vi "Write Teller.vi"(7 "Msg in":refnum<class "Msg.lvclass">, 10 "Teller":T1 {"Absolute Time" format="%<%x %.3X>T"}) -> (5 "Msg out":refnum<class "Msg.lvclass">)   [LabVIEW 2020, in "jettl.lvlib"]
uses:
  jettl.lvlib
  Msg/Msg.lvclass
  Teller Metadata/Teller Metadata.lvclass
  Msg Input/Msg Input.lvclass
  Teller.ctl
  Relation.ctl
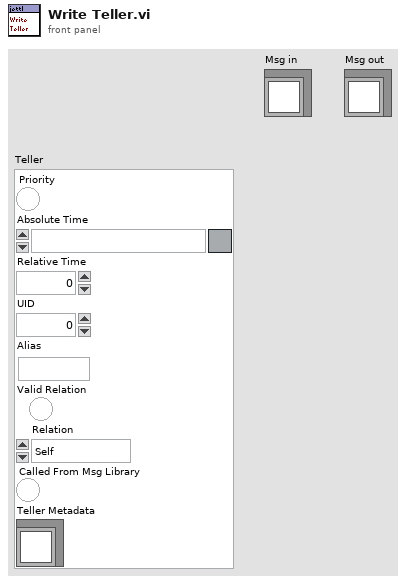
[diagram p1: front panel]
types:
  T1 = typedef "jettl.lvlib/Teller.ctl" = cluster{"Priority":bool, "Absolute Time":timestamp, "Relative Time":dbl, "UID":i32, "Alias":string, "Valid Relation":bool, "Relation":T2, "Called From Msg Library":bool, "Teller Metadata":refnum<class "Teller Metadata.lvclass">}
  T2 = typedef "jettl.lvlib/Relation.ctl" = enum16{"Self", "Parent", "Child"}
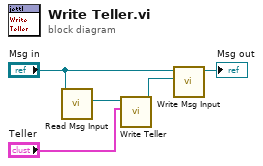
[diagram p0: block diagram]
diagram:
  n1 = call-dynamic "Read Msg Input.vi"("Msg in"="Msg in") -> ("Msg Input"=w3:refnum<class "Msg Input.lvclass">)  [unwired: 10 in]
  n2 = call-dynamic "Write Teller.vi"("Teller"="Teller", "Msg Input in"=w3) -> ("Msg Input out"=w2:refnum<class "Msg Input.lvclass">)  [unwired: 9 in]
  n3 = call-dynamic "Write Msg Input.vi"("Msg Input"=w2, "Msg in"="Msg in") -> ("Msg out"=→"Msg out":refnum<class "Msg.lvclass">)  [unwired: 9 in]
